vi "ADCPro Errors.vi"() -> (0 "Error Description - Custom":string[](array[string]), 1 "Error Codes - Custom":i32[](array[numeric]))   [LabVIEW 2010, in "ErrorLog.lvlib"]
doc: "This VI populates the default error events from the global variables.\n\nInputs:\nGlobal variable\n\nOutputs:\nError Codes - custom: error codes from global variable\nError Description - custom error description from global variable"
uses:
  ErrorLog.lvlib
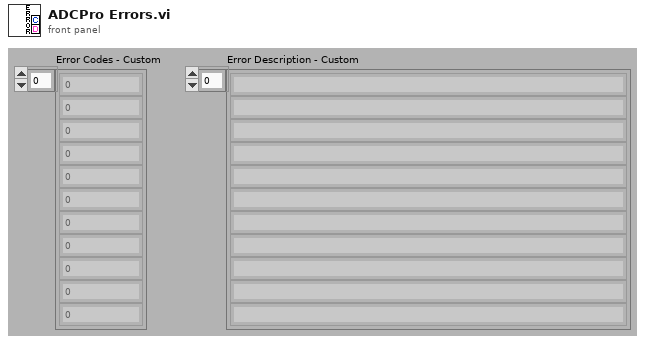
[diagram p1: front panel]
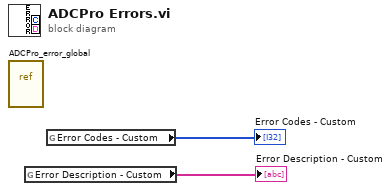
[diagram p0: block diagram]
diagram:
  n1 = vi-ref "ADCPro_error_global.vi"() -> ()  [unwired: 1 out]
  n2 = global read "ADCPro_error_global.vi" "Error Description - Custom"() -> (→"Error Description - Custom":string[])
  n3 = global read "ADCPro_error_global.vi" "Error Codes - Custom"() -> (→"Error Codes - Custom":i32[])
